vi "example_singleRun_stopNotifier.vi"() -> ()   [LabVIEW 2023]
doc: "This example demonstrates the use of TLC_Daemon for launching, controlling, and stopping asynchronous background tasks in a clean, object-oriented manner. It utilizes a boolean notifier mechanism to stop active tasks."
uses:
  Task_BoolStopNotifier/Task_BoolStopNotifier.lvclass
  TaskController/TaskController.lvclass
panel:
  out "loopCounter":i32
  out "isRunning":bool
  # "Example of TaskController with Boolean Notifier Stop Mechanism"
  # "Instruction:\n1. Press RUN button.\n\n2. A single task will run for approximately 5 seconds and then stop:\n    - the isRunning led will be True during task execution.\n    - the loopCounter field shows loopCounter value taken from the task output. \n\nFor details, view code and its comments"
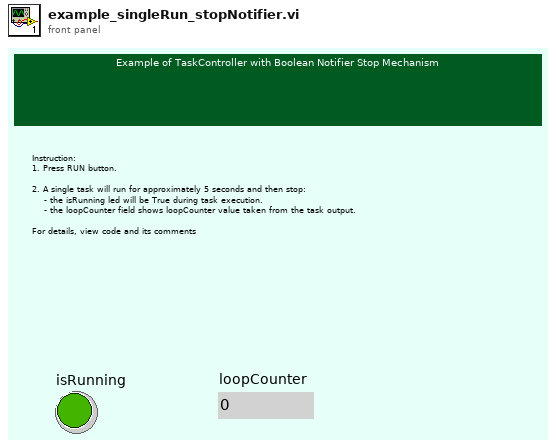
[diagram p1: front panel]
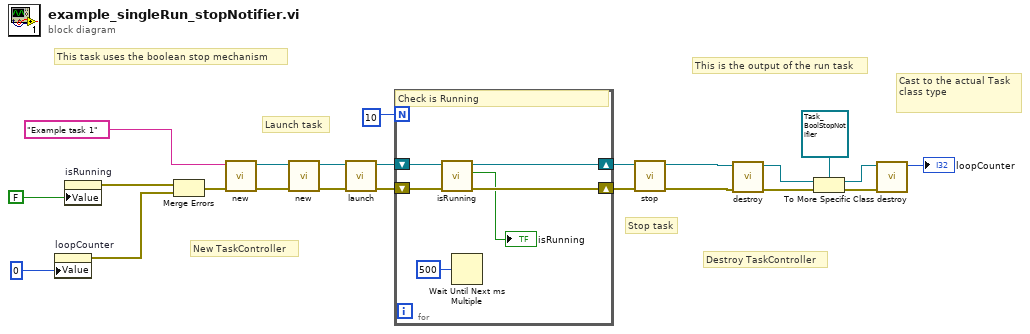
[diagram p0: block diagram]
diagram:
  # "This task uses the boolean stop mechanism"
  # "Cast to the actual Task class type"
  # "This is the output of the run task"
  # "Destroy TaskController"
  # "Stop task"
  # "Launch task"
  # "New TaskController"
  n1 = property on="loopCounter" class="DigNum (strict)"("Value"=0 ("loopCounter")) -> (error out=w4:errorcluster)  [unwired: 2 in, 1 out]
  n2 = property on="isRunning" class="Bool (strict)"("Value"=FALSE ("isRunning")) -> (error out=w3:errorcluster)  [unwired: 2 in, 1 out]
  n3 = Merge Errors(w3, w4) -> (w2:errorcluster)
  n4 = call "new.vi"("error in (no error)"=w2, "description"="Example task 1") -> ("error out"=w23:errorcluster, "ExampleTask_StopNotifier out"=w11:refnum<class "Task_BoolStopNotifier.lvclass">)  [unwired: 8 in]
  n5 = call "new.vi"("error in (no error)"=w23, "task"=w11) -> ("error out"=w21:errorcluster, "TaskController out"=w20:refnum<class "TaskController.lvclass">)  [unwired: 8 in]
  n6 = call "launch.vi"("error in (no error)"=w21, "TaskController in"=w20) -> ("error out"=w19:errorcluster, "TaskController out"=w18:refnum<class "TaskController.lvclass">)  [unwired: 8 in]
  n7 = for {
    N: 10 -> [_]
    shift-right: [w27] -> w15
    shift-left: w18 -> [w28]
    shift-right: [w26] -> w16
    shift-left: w19 -> [w29]
    # "Check is Running"
    n8 = call "isRunning.vi"("error in (no error)"=w29, "TaskController in"=w28) -> ("error out"=w26:errorcluster, "isRunning"=→"isRunning":bool, "TaskController out"=w27:refnum<class "TaskController.lvclass">)  [unwired: 7 in]
    n9 = Wait Until Next ms Multiple(millisecond multiple=u32 500 ("milliseconds to wait")) -> ()  [unwired: 1 out]
  }
  n10 = call "stop.vi"("error in (no error)"=w16, "TaskController in"=w15) -> ("error out"=w14:errorcluster, "TaskController out"=w13:refnum<class "TaskController.lvclass">)  [unwired: 8 in]
  n11 = call "destroy.vi"("error in (no error)"=w14, "TaskController in"=w13) -> ("error out"=w10:errorcluster, "taskResult"=w12:refnum<class "ITask.lvclass">)  [unwired: 7 in, 1 out]
  n12 = To More Specific Class(target class=refnum<class "Task_BoolStopNotifier.lvclass"> refnum ("ExampleTask_StopNotifier out"), reference=w12, error in=w10) -> (specific class reference=w9:refnum<class "Task_BoolStopNotifier.lvclass">, error out=w8:errorcluster)
  n13 = call "destroy.vi"("error in (no error)"=w8, "ExampleTask_StopNotifier in"=w9) -> ("loopCounter"=→"loopCounter":i32)  [unwired: 8 in, 1 out]
